vi "GlobalVariables.vi"() -> ()   [LabVIEW 2011]
uses:
  Controls/PC Cluster.ctl
  Controls/Device Cluster.ctl
  Controls/MFC Cluster.ctl
  Controls/RTPC Cluster.ctl
  Controls/GP275 Cluster.ctl
  Controls/BAR Cluster.ctl
  Controls/EZ-ZONE Input Cluster.ctl
  Controls/EZ-ZONE Output Cluster.ctl
  Controls/GP354 Cluster.ctl
  Controls/DNet StatusRegister Cluster.ctl
  Controls/DNet Status Cluster.ctl
  Controls/DNet CommandRegister Cluster.ctl
  Controls/TurboMotor Response Cluster.ctl
  Controls/TurboMotor Command Cluster.ctl
panel:
  out "Loop Started":bool
  out "Loop Running":bool
  in  "Write Enabled":bool
  in  "Reinitialize?":bool
  in  "Tab Control":T1(tab)
  in  "DNet CommandRegister Buffer":bool[](array[boolean])
  in  "DNet ScanCounter Strings":string[](array[string])
  out "DNet LCD Array":string[](array[string])
  in  "DNet CommandRegister Array":T2[](array[typedef])=[{"Run"=FALSE, "Fault"=FALSE, "DisableNetowrk"=FALSE, "HaltScanner"=FALSE, "Reset"=FALSE}, {"Run"=FALSE, "Fault"=FALSE, "DisableNetowrk"=FALSE, "HaltScanner"=FALSE, "Reset"=FALSE}, {"Run"=FALSE, "Fault"=FALSE, "DisableNetowrk"=FALSE, "HaltScanner"=FALSE, "Reset"=FALSE}, {"Run"=FALSE, "Fault"=FALSE, "DisableNetowrk"=FALSE, "HaltScanner"=FALSE, "Reset"=FALSE}]
  in  "DNet Status Array":T3[](array[typedef])
  out "DNet StatusRegister Array":T4[](array[typedef])
  in  "DNet StatusRegister Strings":string[](array[string])
  in  "DNet Status Strings":string[](array[string])
  in  "DNet CommandRegister Strings":string[](array[string])
  in  "Dnet Input Bytes":u8[](array[numeric])
  out "Dnet Output Bytes":u8[](array[numeric])
  out "Dnet Map Strings":string[][](array[string])=[["Dnet", "Node", "Type", "ID Number", "SCCM", "FullScale", "Input Bytes", "Output Bytes", "Input Start Location", "Output Start Location"], ["A", "1", "MFC", "1", "200", "24576", "8", "2", "0", "0"], ["A", "2", "MFC", "44", "2000", "24576", "8", "2", "8", "2"], ["A", "3", "MFC", "45", "200", "24576", "8", "2", "16", "4"], ["A", "4", "PC", "10", "2000", "0", "8", "2", "24", "6"], ["A", "5", "MFC", "2", "200", "24576", "8", "2", "32", "8"], ["A", "6", "MFC", "46", "2000", "24576", "8", "2", "40", "10"], ["A", "7", "MFC", "47", "200", "24576", "8", "2", "48", "12"], ["A", "8", "PC", "11", "2000", "0", "8", "2", "56", "14"], ["A", "9", "MFC", "3", "1000", "24576", "8", "2", "64", "16"], ["A", "10", "PC", "12", "1000", "0", "8", "2", "72", "18"], ["A", "11", "UNITMFC", "4", "500", "0", "8", "2", "80", "20"], ["A", "12", "PC", "13", "500", "0", "8", "2", "88", "22"], ["A", "13", "MFC", "5", "100", "24576", "8", "2", "96", "24"], ["A", "14", "MFC", "48", "1000", "24576", "8", "2", "104", "26"], ["A", "15", "MFC", "49", "100", "24576", "8", "2", "112", "28"], ["A", "16", "PC", "14", "1000", "0", "8", "2", "120", "30"], ["A", "17", "MFC", "6", "100", "24576", "8", "2", "128", "32"], ["A", "19", "MFC", "51", "100", "24576", "8", "2", "136", "34"], ["A", "20", "PC", "15", "1000", "0", "8", "2", "144", "36"], ["A", "21", "MFC", "7", "100", "24576", "8", "2", "152", "38"], ["A", "23", "MFC", "53", "100", "24576", "8", "2", "160", "40"], ["A", "24", "PC", "16", "1000", "0", "8", "2", "168", "42"], ["A", "25", "MFC", "8", "200", "24576", "8", "2", "176", "44"], ["A", "27", "MFC", "55", "200", "24576", "8", "2", "184", "46"], ["A", "28", "PC", "17", "1000", "0", "8", "2", "192", "48"], ["A", "31", "MFC", "37", "100", "24576", "8", "2", "200", "50"], ["A", "32", "MFC", "56", "500", "24576", "8", "2", "208", "52"], ["A", "37", "MFC", "52", "1000", "24576", "8", "2", "216", "54"], ["A", "42", "MFC", "42", "500", "24576", "8", "2", "224", "56"], ["A", "48", "BAR", "90", "0", "0", "3", "0", "232", "58"], ["A", "49", "RTPC", "29", "5000", "24576", "8", "3", "235", "58"], ["A", "50", "UNITMFC", "50", "1000", "24576", "8", "2", "243", "61"], ["A", "51", "UNITMFC", "54", "2000", "24576", "8", "2", "251", "63"], ["A", "53", "RTPC", "27", "5000", "24576", "8", "3", "259", "65"], ["A", "54", "RTPC", "28", "5000", "24576", "8", "3", "267", "68"], ["A", "55", "MFC", "57", "1000", "24576", "8", "2", "275", "71"], ["A", "56", "MFC", "41", "10", "24576", "8", "2", "283", "73"], ["A", "61", "BAR", "91", "0", "0", "3", "0", "291", "75"], ["B", "1", "MFC", "78", "2000", "24576", "8", "2", "294", "75"], ["B", "2", "MFC", "79", "2000", "24576", "8", "2", "302", "77"], ["B", "3", "MFC", "80", "2000", "24576", "8", "2", "310", "79"], ["B", "4", "MFC", "83", "20000", "24576", "8", "2", "318", "81"], ["B", "5", "MFC", "81", "20000", "24576", "8", "2", "326", "83"], ["B", "6", "MFC", "82", "20000", "24576", "8", "2", "334", "85"], ["B", "8", "MFC", "68", "2000", "24576", "8", "2", "342", "87"], ["B", "9", "MFC", "85", "1000", "24576", "8", "2", "350", "89"], ["B", "10", "MFC", "69", "2000", "24576", "8", "2", "358", "91"], ["B", "11", "MFC", "86", "2000", "24576", "8", "2", "366", "93"], ["B", "12", "MFC", "70", "500", "24576", "8", "2", "374", "95"], ["B", "13", "MFC", "73", "1000", "24576", "8", "2", "382", "97"], ["B", "14", "MFC", "74", "1000", "24576", "8", "2", "390", "99"], ["B", "15", "MFC", "75", "5000", "24576", "8", "2", "398", "101"], ["B", "16", "BAR", "92", "0", "0", "3", "0", "406", "103"], ["B", "21", "GP354", "0", "0", "0", "3", "1", "409", "103"], ["B", "22", "GP275", "0", "0", "0", "5", "0", "412", "104"], ["C", "1", "FESTO", "1", "0", "0", "2", "2", "417", "104"], ["C", "2", "FESTO", "2", "0", "0", "2", "2", "419", "106"], ["C", "3", "FESTO", "3", "0", "0", "2", "2", "421", "108"], ["C", "4", "FESTO", "4", "0", "0", "2", "2", "423", "110"], ["C", "5", "FESTO", "5", "0", "0", "2", "2", "425", "112"], ["C", "6", "FESTO", "6", "0", "0", "2", "2", "427", "114"], ["C", "7", "FESTO", "7", "0", "0", "2", "2", "429", "116"], ["C", "8", "FESTO", "8", "0", "0", "2", "2", "431", "118"]]
  in  "Dnet Input Strings":string[](array[string])=["Dnet_A_N01_POL_I.Data", "Dnet_A_N01_POL_I.Data1", "Dnet_A_N01_POL_I.Data2", "Dnet_A_N01_POL_I.ExtendedData", "Dnet_A_N01_POL_I.ExtendedData1", "Dnet_A_N01_POL_I.ExtendedData2", "Dnet_A_N01_POL_I.ExtendedData3", "Dnet_A_N01_POL_I.ExtendedData4", "Dnet_A_N02_POL_I.Data", "Dnet_A_N02_POL_I.Data1", "Dnet_A_N02_POL_I.Data2", "Dnet_A_N02_POL_I.ExtendedData", "Dnet_A_N02_POL_I.ExtendedData1", "Dnet_A_N02_POL_I.ExtendedData2", "Dnet_A_N02_POL_I.ExtendedData3", "Dnet_A_N02_POL_I.ExtendedData4", "Dnet_A_N03_POL_I.Data", "Dnet_A_N03_POL_I.Data1", "Dnet_A_N03_POL_I.Data2", "Dnet_A_N03_POL_I.ExtendedData", "Dnet_A_N03_POL_I.ExtendedData1", "Dnet_A_N03_POL_I.ExtendedData2", "Dnet_A_N03_POL_I.ExtendedData3", "Dnet_A_N03_POL_I.ExtendedData4", "Dnet_A_N04_POL_I.Data", "Dnet_A_N04_POL_I.Data1", "Dnet_A_N04_POL_I.Data2", "Dnet_A_N04_POL_I.ExtendedData", "Dnet_A_N04_POL_I.ExtendedData1", "Dnet_A_N04_POL_I.ExtendedData2", "Dnet_A_N04_POL_I.ExtendedData3", "Dnet_A_N04_POL_I.ExtendedData4", "Dnet_A_N05_POL_I.Data", "Dnet_A_N05_POL_I.Data1", "Dnet_A_N05_POL_I.Data2", "Dnet_A_N05_POL_I.ExtendedData", "Dnet_A_N05_POL_I.ExtendedData1", "Dnet_A_N05_POL_I.ExtendedData2", "Dnet_A_N05_POL_I.ExtendedData3", "Dnet_A_N05_POL_I.ExtendedData4", "Dnet_A_N06_POL_I.Data", "Dnet_A_N06_POL_I.Data1", "Dnet_A_N06_POL_I.Data2", "Dnet_A_N06_POL_I.ExtendedData", "Dnet_A_N06_POL_I.ExtendedData1", "Dnet_A_N06_POL_I.ExtendedData2", "Dnet_A_N06_POL_I.ExtendedData3", "Dnet_A_N06_POL_I.ExtendedData4", "Dnet_A_N07_POL_I.Data", "Dnet_A_N07_POL_I.Data1", "Dnet_A_N07_POL_I.Data2", "Dnet_A_N07_POL_I.ExtendedData", "Dnet_A_N07_POL_I.ExtendedData1", "Dnet_A_N07_POL_I.ExtendedData2", "Dnet_A_N07_POL_I.ExtendedData3", "Dnet_A_N07_POL_I.ExtendedData4", "Dnet_A_N08_POL_I.Data", "Dnet_A_N08_POL_I.Data1", "Dnet_A_N08_POL_I.Data2", "Dnet_A_N08_POL_I.ExtendedData", "Dnet_A_N08_POL_I.ExtendedData1", "Dnet_A_N08_POL_I.ExtendedData2", "Dnet_A_N08_POL_I.ExtendedData3", "Dnet_A_N08_POL_I.ExtendedData4", "Dnet_A_N09_POL_I.Data", "Dnet_A_N09_POL_I.Data1", "Dnet_A_N09_POL_I.Data2", "Dnet_A_N09_POL_I.ExtendedData", "Dnet_A_N09_POL_I.ExtendedData1", "Dnet_A_N09_POL_I.ExtendedData2", "Dnet_A_N09_POL_I.ExtendedData3", "Dnet_A_N09_POL_I.ExtendedData4", "Dnet_A_N10_POL_I.Data", "Dnet_A_N10_POL_I.Data1", "Dnet_A_N10_POL_I.Data2", "Dnet_A_N10_POL_I.ExtendedData", "Dnet_A_N10_POL_I.ExtendedData1", "Dnet_A_N10_POL_I.ExtendedData2", "Dnet_A_N10_POL_I.ExtendedData3", "Dnet_A_N10_POL_I.ExtendedData4", "Dnet_A_N11_POL_I.Data_x.Data_0", "Dnet_A_N11_POL_I.Data_x.Data_1", "Dnet_A_N11_POL_I.Data_x.Data_2", "Dnet_A_N11_POL_I.Data_x.Data_3", "Dnet_A_N11_POL_I.Data_x.Data_4", "Dnet_A_N11_POL_I.Data_x.Data_5", "Dnet_A_N11_POL_I.Data_x.Data_6", "Dnet_A_N11_POL_I.Data_x.Data_7", "Dnet_A_N12_POL_I.Data", "Dnet_A_N12_POL_I.Data1", "Dnet_A_N12_POL_I.Data2", "Dnet_A_N12_POL_I.ExtendedData", "Dnet_A_N12_POL_I.ExtendedData1", "Dnet_A_N12_POL_I.ExtendedData2", "Dnet_A_N12_POL_I.ExtendedData3", "Dnet_A_N12_POL_I.ExtendedData4", "Dnet_A_N13_POL_I.Data", "Dnet_A_N13_POL_I.Data1", "Dnet_A_N13_POL_I.Data2", "Dnet_A_N13_POL_I.ExtendedData", "Dnet_A_N13_POL_I.ExtendedData1", "Dnet_A_N13_POL_I.ExtendedData2", "Dnet_A_N13_POL_I.ExtendedData3", "Dnet_A_N13_POL_I.ExtendedData4", "Dnet_A_N14_POL_I.Data", "Dnet_A_N14_POL_I.Data1", "Dnet_A_N14_POL_I.Data2", "Dnet_A_N14_POL_I.ExtendedData", "Dnet_A_N14_POL_I.ExtendedData1", "Dnet_A_N14_POL_I.ExtendedData2", "Dnet_A_N14_POL_I.ExtendedData3", "Dnet_A_N14_POL_I.ExtendedData4", "Dnet_A_N15_POL_I.Data", "Dnet_A_N15_POL_I.Data1", "Dnet_A_N15_POL_I.Data2", "Dnet_A_N15_POL_I.ExtendedData", "Dnet_A_N15_POL_I.ExtendedData1", "Dnet_A_N15_POL_I.ExtendedData2", "Dnet_A_N15_POL_I.ExtendedData3", "Dnet_A_N15_POL_I.ExtendedData4", "Dnet_A_N16_POL_I.Data", "Dnet_A_N16_POL_I.Data1", "Dnet_A_N16_POL_I.Data2", "Dnet_A_N16_POL_I.ExtendedData", "Dnet_A_N16_POL_I.ExtendedData1", "Dnet_A_N16_POL_I.ExtendedData2", "Dnet_A_N16_POL_I.ExtendedData3", "Dnet_A_N16_POL_I.ExtendedData4", "Dnet_A_N17_POL_I.Data", "Dnet_A_N17_POL_I.Data1", "Dnet_A_N17_POL_I.Data2", "Dnet_A_N17_POL_I.ExtendedData", "Dnet_A_N17_POL_I.ExtendedData1", "Dnet_A_N17_POL_I.ExtendedData2", "Dnet_A_N17_POL_I.ExtendedData3", "Dnet_A_N17_POL_I.ExtendedData4", "Dnet_A_N19_POL_I.Data", "Dnet_A_N19_POL_I.Data1", "Dnet_A_N19_POL_I.Data2", "Dnet_A_N19_POL_I.ExtendedData", "Dnet_A_N19_POL_I.ExtendedData1", "Dnet_A_N19_POL_I.ExtendedData2", "Dnet_A_N19_POL_I.ExtendedData3", "Dnet_A_N19_POL_I.ExtendedData4", "Dnet_A_N20_POL_I.Data", "Dnet_A_N20_POL_I.Data1", "Dnet_A_N20_POL_I.Data2", "Dnet_A_N20_POL_I.ExtendedData", "Dnet_A_N20_POL_I.ExtendedData1", "Dnet_A_N20_POL_I.ExtendedData2", "Dnet_A_N20_POL_I.ExtendedData3", "Dnet_A_N20_POL_I.ExtendedData4", "Dnet_A_N21_POL_I.Data", "Dnet_A_N21_POL_I.Data1", "Dnet_A_N21_POL_I.Data2", "Dnet_A_N21_POL_I.ExtendedData", "Dnet_A_N21_POL_I.ExtendedData1", "Dnet_A_N21_POL_I.ExtendedData2", "Dnet_A_N21_POL_I.ExtendedData3", "Dnet_A_N21_POL_I.ExtendedData4", "Dnet_A_N23_POL_I.Data", "Dnet_A_N23_POL_I.Data1", "Dnet_A_N23_POL_I.Data2", "Dnet_A_N23_POL_I.ExtendedData", "Dnet_A_N23_POL_I.ExtendedData1", "Dnet_A_N23_POL_I.ExtendedData2", "Dnet_A_N23_POL_I.ExtendedData3", "Dnet_A_N23_POL_I.ExtendedData4", "Dnet_A_N24_POL_I.Data", "Dnet_A_N24_POL_I.Data1", "Dnet_A_N24_POL_I.Data2", "Dnet_A_N24_POL_I.ExtendedData", "Dnet_A_N24_POL_I.ExtendedData1", "Dnet_A_N24_POL_I.ExtendedData2", "Dnet_A_N24_POL_I.ExtendedData3", "Dnet_A_N24_POL_I.ExtendedData4", "Dnet_A_N25_POL_I.Data", "Dnet_A_N25_POL_I.Data1", "Dnet_A_N25_POL_I.Data2", "Dnet_A_N25_POL_I.ExtendedData", "Dnet_A_N25_POL_I.ExtendedData1", "Dnet_A_N25_POL_I.ExtendedData2", "Dnet_A_N25_POL_I.ExtendedData3", "Dnet_A_N25_POL_I.ExtendedData4", "Dnet_A_N27_POL_I.Data", "Dnet_A_N27_POL_I.Data1", "Dnet_A_N27_POL_I.Data2", "Dnet_A_N27_POL_I.ExtendedData", "Dnet_A_N27_POL_I.ExtendedData1", "Dnet_A_N27_POL_I.ExtendedData2", "Dnet_A_N27_POL_I.ExtendedData3", "Dnet_A_N27_POL_I.ExtendedData4", "Dnet_A_N28_POL_I.Data", "Dnet_A_N28_POL_I.Data1", "Dnet_A_N28_POL_I.Data2", "Dnet_A_N28_POL_I.ExtendedData", "Dnet_A_N28_POL_I.ExtendedData1", "Dnet_A_N28_POL_I.ExtendedData2", "Dnet_A_N28_POL_I.ExtendedData3", "Dnet_A_N28_POL_I.ExtendedData4", "Dnet_A_N31_POL_I.Data", "Dnet_A_N31_POL_I.Data1", "Dnet_A_N31_POL_I.Data2", "Dnet_A_N31_POL_I.ExtendedData", "Dnet_A_N31_POL_I.ExtendedData1", "Dnet_A_N31_POL_I.ExtendedData2", "Dnet_A_N31_POL_I.ExtendedData3", "Dnet_A_N31_POL_I.ExtendedData4", "Dnet_A_N32_POL_I.Data", "Dnet_A_N32_POL_I.Data1", "Dnet_A_N32_POL_I.Data2", "Dnet_A_N32_POL_I.ExtendedData", "Dnet_A_N32_POL_I.ExtendedData1", "Dnet_A_N32_POL_I.ExtendedData2", "Dnet_A_N32_POL_I.ExtendedData3", "Dnet_A_N32_POL_I.ExtendedData4", "Dnet_A_N37_POL_I.Data_x.Data_0", "Dnet_A_N37_POL_I.Data_x.Data_1", "Dnet_A_N37_POL_I.Data_x.Data_2", "Dnet_A_N37_POL_I.Data_x.Data_3", "Dnet_A_N37_POL_I.Data_x.Data_4", "Dnet_A_N37_POL_I.Data_x.Data_5", "Dnet_A_N37_POL_I.Data_x.Data_6", "Dnet_A_N37_POL_I.Data_x.Data_7", "Dnet_A_N42_POL_I.Data", "Dnet_A_N42_POL_I.Data1", "Dnet_A_N42_POL_I.Data2", "Dnet_A_N42_POL_I.ExtendedData", "Dnet_A_N42_POL_I.ExtendedData1", "Dnet_A_N42_POL_I.ExtendedData2", "Dnet_A_N42_POL_I.ExtendedData3", "Dnet_A_N42_POL_I.ExtendedData4", "Dnet_A_N48_POL_I.Data_x.Data_0", "Dnet_A_N48_POL_I.Data_x.Data_1", "Dnet_A_N48_POL_I.Data_x.Data_2", "Dnet_A_N49_POL_I.Data", "Dnet_A_N49_POL_I.Data1", "Dnet_A_N49_POL_I.Data2", "Dnet_A_N49_POL_I.ExtendedData", "Dnet_A_N49_POL_I.ExtendedData1", "Dnet_A_N49_POL_I.ExtendedData2", "Dnet_A_N49_POL_I.ExtendedData3", "Dnet_A_N49_POL_I.ExtendedData4", "Dnet_A_N50_POL_I.Data_x.Data_0", "Dnet_A_N50_POL_I.Data_x.Data_1", "Dnet_A_N50_POL_I.Data_x.Data_2", "Dnet_A_N50_POL_I.Data_x.Data_3", "Dnet_A_N50_POL_I.Data_x.Data_4", "Dnet_A_N50_POL_I.Data_x.Data_5", "Dnet_A_N50_POL_I.Data_x.Data_6", "Dnet_A_N50_POL_I.Data_x.Data_7", "Dnet_A_N51_POL_I.Data_x.Data_0", "Dnet_A_N51_POL_I.Data_x.Data_1", "Dnet_A_N51_POL_I.Data_x.Data_2", "Dnet_A_N51_POL_I.Data_x.Data_3", "Dnet_A_N51_POL_I.Data_x.Data_4", "Dnet_A_N51_POL_I.Data_x.Data_5", "Dnet_A_N51_POL_I.Data_x.Data_6", "Dnet_A_N51_POL_I.Data_x.Data_7", "Dnet_A_N53_POL_I.Data", "Dnet_A_N53_POL_I.Data1", "Dnet_A_N53_POL_I.Data2", "Dnet_A_N53_POL_I.ExtendedData", "Dnet_A_N53_POL_I.ExtendedData1", "Dnet_A_N53_POL_I.ExtendedData2", "Dnet_A_N53_POL_I.ExtendedData3", "Dnet_A_N53_POL_I.ExtendedData4", "Dnet_A_N54_POL_I.Data", "Dnet_A_N54_POL_I.Data1", "Dnet_A_N54_POL_I.Data2", "Dnet_A_N54_POL_I.ExtendedData", "Dnet_A_N54_POL_I.ExtendedData1", "Dnet_A_N54_POL_I.ExtendedData2", "Dnet_A_N54_POL_I.ExtendedData3", "Dnet_A_N54_POL_I.ExtendedData4", "Dnet_A_N55_POL_I.Data", "Dnet_A_N55_POL_I.Data1", "Dnet_A_N55_POL_I.Data2", "Dnet_A_N55_POL_I.ExtendedData", "Dnet_A_N55_POL_I.ExtendedData1", "Dnet_A_N55_POL_I.ExtendedData2", "Dnet_A_N55_POL_I.ExtendedData3", "Dnet_A_N55_POL_I.ExtendedData4", "Dnet_A_N56_POL_I.Data", "Dnet_A_N56_POL_I.Data1", "Dnet_A_N56_POL_I.Data2", "Dnet_A_N56_POL_I.ExtendedData", "Dnet_A_N56_POL_I.ExtendedData1", "Dnet_A_N56_POL_I.ExtendedData2", "Dnet_A_N56_POL_I.ExtendedData3", "Dnet_A_N56_POL_I.ExtendedData4", "Dnet_A_N61_POL_I.Data_x.Data_0", "Dnet_A_N61_POL_I.Data_x.Data_1", "Dnet_A_N61_POL_I.Data_x.Data_2", "Dnet_B_N01_POL_I.Data", "Dnet_B_N01_POL_I.Data1", "Dnet_B_N01_POL_I.Data2", "Dnet_B_N01_POL_I.ExtendedData", "Dnet_B_N01_POL_I.ExtendedData1", "Dnet_B_N01_POL_I.ExtendedData2", "Dnet_B_N01_POL_I.ExtendedData3", "Dnet_B_N01_POL_I.ExtendedData4", "Dnet_B_N02_POL_I.Data", "Dnet_B_N02_POL_I.Data1", "Dnet_B_N02_POL_I.Data2", "Dnet_B_N02_POL_I.ExtendedData", "Dnet_B_N02_POL_I.ExtendedData1", "Dnet_B_N02_POL_I.ExtendedData2", "Dnet_B_N02_POL_I.ExtendedData3", "Dnet_B_N02_POL_I.ExtendedData4", "Dnet_B_N03_POL_I.Data", "Dnet_B_N03_POL_I.Data1", "Dnet_B_N03_POL_I.Data2", "Dnet_B_N03_POL_I.ExtendedData", "Dnet_B_N03_POL_I.ExtendedData1", "Dnet_B_N03_POL_I.ExtendedData2", "Dnet_B_N03_POL_I.ExtendedData3", "Dnet_B_N03_POL_I.ExtendedData4", "Dnet_B_N04_POL_I.Data", "Dnet_B_N04_POL_I.Data1", "Dnet_B_N04_POL_I.Data2", "Dnet_B_N04_POL_I.ExtendedData", "Dnet_B_N04_POL_I.ExtendedData1", "Dnet_B_N04_POL_I.ExtendedData2", "Dnet_B_N04_POL_I.ExtendedData3", "Dnet_B_N04_POL_I.ExtendedData4", "Dnet_B_N05_POL_I.Data", "Dnet_B_N05_POL_I.Data1", "Dnet_B_N05_POL_I.Data2", "Dnet_B_N05_POL_I.ExtendedData", "Dnet_B_N05_POL_I.ExtendedData1", "Dnet_B_N05_POL_I.ExtendedData2", "Dnet_B_N05_POL_I.ExtendedData3", "Dnet_B_N05_POL_I.ExtendedData4", "Dnet_B_N06_POL_I.Data", "Dnet_B_N06_POL_I.Data1", "Dnet_B_N06_POL_I.Data2", "Dnet_B_N06_POL_I.ExtendedData", "Dnet_B_N06_POL_I.ExtendedData1", "Dnet_B_N06_POL_I.ExtendedData2", "Dnet_B_N06_POL_I.ExtendedData3", "Dnet_B_N06_POL_I.ExtendedData4", "Dnet_B_N08_POL_I.Data", "Dnet_B_N08_POL_I.Data1", "Dnet_B_N08_POL_I.Data2", "Dnet_B_N08_POL_I.ExtendedData", "Dnet_B_N08_POL_I.ExtendedData1", "Dnet_B_N08_POL_I.ExtendedData2", "Dnet_B_N08_POL_I.ExtendedData3", "Dnet_B_N08_POL_I.ExtendedData4", "Dnet_B_N09_POL_I.Data", "Dnet_B_N09_POL_I.Data1", "Dnet_B_N09_POL_I.Data2", "Dnet_B_N09_POL_I.ExtendedData", "Dnet_B_N09_POL_I.ExtendedData1", "Dnet_B_N09_POL_I.ExtendedData2", "Dnet_B_N09_POL_I.ExtendedData3", "Dnet_B_N09_POL_I.ExtendedData4", "Dnet_B_N10_POL_I.Data", "Dnet_B_N10_POL_I.Data1", "Dnet_B_N10_POL_I.Data2", "Dnet_B_N10_POL_I.ExtendedData", "Dnet_B_N10_POL_I.ExtendedData1", "Dnet_B_N10_POL_I.ExtendedData2", "Dnet_B_N10_POL_I.ExtendedData3", "Dnet_B_N10_POL_I.ExtendedData4", "Dnet_B_N11_POL_I.Data", "Dnet_B_N11_POL_I.Data1", "Dnet_B_N11_POL_I.Data2", "Dnet_B_N11_POL_I.ExtendedData", "Dnet_B_N11_POL_I.ExtendedData1", "Dnet_B_N11_POL_I.ExtendedData2", "Dnet_B_N11_POL_I.ExtendedData3", "Dnet_B_N11_POL_I.ExtendedData4", "Dnet_B_N12_POL_I.Data", "Dnet_B_N12_POL_I.Data1", "Dnet_B_N12_POL_I.Data2", "Dnet_B_N12_POL_I.ExtendedData", "Dnet_B_N12_POL_I.ExtendedData1", "Dnet_B_N12_POL_I.ExtendedData2", "Dnet_B_N12_POL_I.ExtendedData3", "Dnet_B_N12_POL_I.ExtendedData4", "Dnet_B_N13_POL_I.Data", "Dnet_B_N13_POL_I.Data1", "Dnet_B_N13_POL_I.Data2", "Dnet_B_N13_POL_I.ExtendedData", "Dnet_B_N13_POL_I.ExtendedData1", "Dnet_B_N13_POL_I.ExtendedData2", "Dnet_B_N13_POL_I.ExtendedData3", "Dnet_B_N13_POL_I.ExtendedData4", "Dnet_B_N14_POL_I.Data", "Dnet_B_N14_POL_I.Data1", "Dnet_B_N14_POL_I.Data2", "Dnet_B_N14_POL_I.ExtendedData", "Dnet_B_N14_POL_I.ExtendedData1", "Dnet_B_N14_POL_I.ExtendedData2", "Dnet_B_N14_POL_I.ExtendedData3", "Dnet_B_N14_POL_I.ExtendedData4", "Dnet_B_N15_POL_I.Data", "Dnet_B_N15_POL_I.Data1", "Dnet_B_N15_POL_I.Data2", "Dnet_B_N15_POL_I.ExtendedData", "Dnet_B_N15_POL_I.ExtendedData1", "Dnet_B_N15_POL_I.ExtendedData2", "Dnet_B_N15_POL_I.ExtendedData3", "Dnet_B_N15_POL_I.ExtendedData4", "Dnet_B_N16_POL_I.Data_x.Data_0", "Dnet_B_N16_POL_I.Data_x.Data_1", "Dnet_B_N16_POL_I.Data_x.Data_2", "Dnet_B_N21_POL_I.Data_x.Data_0", "Dnet_B_N21_POL_I.Data_x.Data_1", "Dnet_B_N21_POL_I.Data_x.Data_2", "Dnet_B_N22_POL_I.Data_x.Data_0", "Dnet_B_N22_POL_I.Data_x.Data_1", "Dnet_B_N22_POL_I.Data_x.Data_2", "Dnet_B_N22_POL_I.Data_x.Data_3", "Dnet_B_N22_POL_I.Data_x.Data_4", "Dnet_C_N01_POL_I.Data", "Dnet_C_N01_STB_I.Data", "Dnet_C_N02_POL_I.Data_x.Data_0", "Dnet_C_N02_POL_I.Data_x.Data_1", "Dnet_C_N03_POL_I.Data_x.Data_0", "Dnet_C_N03_POL_I.Data_x.Data_1", "Dnet_C_N04_POL_I.Data_x.Data_0", "Dnet_C_N04_POL_I.Data_x.Data_1", "Dnet_C_N05_POL_I.Data_x.Data_0", "Dnet_C_N05_POL_I.Data_x.Data_1", "Dnet_C_N06_POL_I.Data_x.Data_0", "Dnet_C_N06_POL_I.Data_x.Data_1", "Dnet_C_N07_POL_I.Data_x.Data_0", "Dnet_C_N07_POL_I.Data_x.Data_1", "Dnet_C_N08_POL_I.Data_x.Data_0", "Dnet_C_N08_POL_I.Data_x.Data_1"]
  in  "Dnet Output Strings":string[](array[string])=["Dnet_A_N01_POL_O.Data_x.Data_0", "Dnet_A_N01_POL_O.Data_x.Data_1", "Dnet_A_N02_POL_O.Data_x.Data_0", "Dnet_A_N02_POL_O.Data_x.Data_1", "Dnet_A_N03_POL_O.Data_x.Data_0", "Dnet_A_N03_POL_O.Data_x.Data_1", "Dnet_A_N04_POL_O.Data_x.Data_0", "Dnet_A_N04_POL_O.Data_x.Data_1", "Dnet_A_N05_POL_O.Data_x.Data_0", "Dnet_A_N05_POL_O.Data_x.Data_1", "Dnet_A_N06_POL_O.Data_x.Data_0", "Dnet_A_N06_POL_O.Data_x.Data_1", "Dnet_A_N07_POL_O.Data_x.Data_0", "Dnet_A_N07_POL_O.Data_x.Data_1", "Dnet_A_N08_POL_O.Data_x.Data_0", "Dnet_A_N08_POL_O.Data_x.Data_1", "Dnet_A_N09_POL_O.Data_x.Data_0", "Dnet_A_N09_POL_O.Data_x.Data_1", "Dnet_A_N10_POL_O.Data_x.Data_0", "Dnet_A_N10_POL_O.Data_x.Data_1", "Dnet_A_N11_POL_O.Data_x.Data_0", "Dnet_A_N11_POL_O.Data_x.Data_1", "Dnet_A_N12_POL_O.Data_x.Data_0", "Dnet_A_N12_POL_O.Data_x.Data_1", "Dnet_A_N13_POL_O.Data_x.Data_0", "Dnet_A_N13_POL_O.Data_x.Data_1", "Dnet_A_N14_POL_O.Data_x.Data_0", "Dnet_A_N14_POL_O.Data_x.Data_1", "Dnet_A_N15_POL_O.Data_x.Data_0", "Dnet_A_N15_POL_O.Data_x.Data_1", "Dnet_A_N16_POL_O.Data_x.Data_0", "Dnet_A_N16_POL_O.Data_x.Data_1", "Dnet_A_N17_POL_O.Data_x.Data_0", "Dnet_A_N17_POL_O.Data_x.Data_1", "Dnet_A_N19_POL_O.Data_x.Data_0", "Dnet_A_N19_POL_O.Data_x.Data_1", "Dnet_A_N20_POL_O.Data_x.Data_0", "Dnet_A_N20_POL_O.Data_x.Data_1", "Dnet_A_N21_POL_O.Data_x.Data_0", "Dnet_A_N21_POL_O.Data_x.Data_1", "Dnet_A_N23_POL_O.Data_x.Data_0", "Dnet_A_N23_POL_O.Data_x.Data_1", "Dnet_A_N24_POL_O.Data_x.Data_0", "Dnet_A_N24_POL_O.Data_x.Data_1", "Dnet_A_N25_POL_O.Data_x.Data_0", "Dnet_A_N25_POL_O.Data_x.Data_1", "Dnet_A_N27_POL_O.Data_x.Data_0", "Dnet_A_N27_POL_O.Data_x.Data_1", "Dnet_A_N28_POL_O.Data_x.Data_0", "Dnet_A_N28_POL_O.Data_x.Data_1", "Dnet_A_N31_POL_O.Data_x.Data_0", "Dnet_A_N31_POL_O.Data_x.Data_1", "Dnet_A_N32_POL_O.Data_x.Data_0", "Dnet_A_N32_POL_O.Data_x.Data_1", "Dnet_A_N37_POL_O.Data_x.Data_0", "Dnet_A_N37_POL_O.Data_x.Data_1", "Dnet_A_N42_POL_O.Data_x.Data_0", "Dnet_A_N42_POL_O.Data_x.Data_1", "Dnet_A_N49_POL_O.Data", "Dnet_A_N49_POL_O.Data1", "Dnet_A_N49_POL_O.ExtendedData", "Dnet_A_N50_POL_O.Data_x.Data_0", "Dnet_A_N50_POL_O.Data_x.Data_1", "Dnet_A_N51_POL_O.Data_x.Data_0", "Dnet_A_N51_POL_O.Data_x.Data_1", "Dnet_A_N53_POL_O.Data", "Dnet_A_N53_POL_O.Data1", "Dnet_A_N53_POL_O.ExtendedData", "Dnet_A_N54_POL_O.Data", "Dnet_A_N54_POL_O.Data1", "Dnet_A_N54_POL_O.ExtendedData", "Dnet_A_N55_POL_O.Data_x.Data_0", "Dnet_A_N55_POL_O.Data_x.Data_1", "Dnet_A_N56_POL_O.Data_x.Data_0", "Dnet_A_N56_POL_O.Data_x.Data_1", "Dnet_B_N01_POL_O.Data_x.Data_0", "Dnet_B_N01_POL_O.Data_x.Data_1", "Dnet_B_N02_POL_O.Data_x.Data_0", "Dnet_B_N02_POL_O.Data_x.Data_1", "Dnet_B_N03_POL_O.Data_x.Data_0", "Dnet_B_N03_POL_O.Data_x.Data_1", "Dnet_B_N04_POL_O.Data_x.Data_0", "Dnet_B_N04_POL_O.Data_x.Data_1", "Dnet_B_N05_POL_O.Data_x.Data_0", "Dnet_B_N05_POL_O.Data_x.Data_1", "Dnet_B_N06_POL_O.Data_x.Data_0", "Dnet_B_N06_POL_O.Data_x.Data_1", "Dnet_B_N08_POL_O.Data_x.Data_0", "Dnet_B_N08_POL_O.Data_x.Data_1", "Dnet_B_N09_POL_O.Data_x.Data_0", "Dnet_B_N09_POL_O.Data_x.Data_1", "Dnet_B_N10_POL_O.Data_x.Data_0", "Dnet_B_N10_POL_O.Data_x.Data_1", "Dnet_B_N11_POL_O.Data_x.Data_0", "Dnet_B_N11_POL_O.Data_x.Data_1", "Dnet_B_N12_POL_O.Data_x.Data_0", "Dnet_B_N12_POL_O.Data_x.Data_1", "Dnet_B_N13_POL_O.Data_x.Data_0", "Dnet_B_N13_POL_O.Data_x.Data_1", "Dnet_B_N14_POL_O.Data_x.Data_0", "Dnet_B_N14_POL_O.Data_x.Data_1", "Dnet_B_N15_POL_O.Data_x.Data_0", "Dnet_B_N15_POL_O.Data_x.Data_1", "Dnet_B_N21_POL_O.Data", "Dnet_C_N01_POL_O.Data_x.Data_0", "Dnet_C_N01_POL_O.Data_x.Data_1", "Dnet_C_N02_POL_O.Data_x.Data_0", "Dnet_C_N02_POL_O.Data_x.Data_1", "Dnet_C_N03_POL_O.Data_x.Data_0", "Dnet_C_N03_POL_O.Data_x.Data_1", "Dnet_C_N04_POL_O.Data_x.Data_0", "Dnet_C_N04_POL_O.Data_x.Data_1", "Dnet_C_N05_POL_O.Data_x.Data_0", "Dnet_C_N05_POL_O.Data_x.Data_1", "Dnet_C_N06_POL_O.Data_x.Data_0", "Dnet_C_N06_POL_O.Data_x.Data_1", "Dnet_C_N07_POL_O.Data_x.Data_0", "Dnet_C_N07_POL_O.Data_x.Data_1", "Dnet_C_N08_POL_O.Data_x.Data_0", "Dnet_C_N08_POL_O.Data_x.Data_1"]
  in  "Ain":dbl[](array[numeric])
  in  "Aout":i16[](array[numeric])
  in  "Ain1 Strings":string[](array[string])=["Local_5_I.Ch0Data", "Local_5_I.Ch1Data", "Local_5_I.Ch2Data", "Local_5_I.Ch3Data", "Local_5_I.Ch4Data", "Local_5_I.Ch5Data", "Local_5_I.Ch6Data", "Local_5_I.Ch7Data", "Local_5_I.Ch8Data", "Local_5_I.Ch9Data", "Local_5_I.Ch10Data", "Local_5_I.Ch11Data", "Local_5_I.Ch12Data", "Local_5_I.Ch13Data", "Local_5_I.Ch14Data", "Local_5_I.Ch15Data"]
  in  "Ain2 Strings":string[](array[string])=["Local_6_I.Ch0Data", "Local_6_I.Ch1Data", "Local_6_I.Ch2Data", "Local_6_I.Ch3Data", "Local_6_I.Ch4Data", "Local_6_I.Ch5Data", "Local_6_I.Ch6Data", "Local_6_I.Ch7Data", "Local_6_I.Ch8Data", "Local_6_I.Ch9Data", "Local_6_I.Ch10Data", "Local_6_I.Ch11Data", "Local_6_I.Ch12Data", "Local_6_I.Ch13Data", "Local_6_I.Ch14Data", "Local_6_I.Ch15Data"]
  in  "Dout Strings":string[](array[string])=["Local_10_O.Data"]
  in  "Din Strings":string[](array[string])=["Local_8_I.Data", "Local_9_I.Data", "Local_10_I.Data"]
  in  "Din1":bool[](array[boolean])=[FALSE, FALSE, FALSE, FALSE, FALSE, FALSE, FALSE, FALSE, FALSE, FALSE, FALSE, FALSE, FALSE, FALSE, FALSE, FALSE, FALSE, FALSE, FALSE, FALSE, FALSE, FALSE, FALSE, FALSE, FALSE, FALSE, FALSE, FALSE, FALSE, FALSE, FALSE, FALSE]
  in  "Dout":bool[](array[boolean])=[FALSE, FALSE, FALSE, FALSE, FALSE, FALSE, FALSE, FALSE, FALSE, FALSE, FALSE, FALSE, FALSE, FALSE, FALSE, FALSE, FALSE, FALSE, FALSE, FALSE, FALSE, FALSE, FALSE, FALSE, FALSE, FALSE, FALSE, FALSE, FALSE, FALSE, FALSE, FALSE]
  in  "Din2":bool[](array[boolean])=[FALSE, FALSE, FALSE, FALSE, FALSE, FALSE, FALSE, FALSE, FALSE, FALSE, FALSE, FALSE, FALSE, FALSE, FALSE, FALSE, FALSE, FALSE, FALSE, FALSE, FALSE, FALSE, FALSE, FALSE, FALSE, FALSE, FALSE, FALSE, FALSE, FALSE, FALSE, FALSE]
  in  "Valve Strings 2":string[](array[string])=["Valve_x.Valve_000", "Valve_x.Valve_001", "Valve_x.Valve_002", "Valve_x.Valve_003", "Valve_x.Valve_004", "Valve_x.Valve_005", "Valve_x.Valve_006", "Valve_x.Valve_007", "Valve_x.Valve_008", "Valve_x.Valve_009", "Valve_x.Valve_010", "Valve_x.Valve_011", "Valve_x.Valve_012", "Valve_x.Valve_013", "Valve_x.Valve_014", "Valve_x.Valve_015", "Valve_x.Valve_016", "Valve_x.Valve_017", "Valve_x.Valve_018", "Valve_x.Valve_019", "Valve_x.Valve_020", "Valve_x.Valve_021", "Valve_x.Valve_022", "Valve_x.Valve_023", "Valve_x.Valve_024", "Valve_x.Valve_025", "Valve_x.Valve_026", "Valve_x.Valve_027", "Valve_x.Valve_028", "Valve_x.Valve_029", "Valve_x.Valve_030", "Valve_x.Valve_031", "Valve_x.Valve_032", "Valve_x.Valve_033", "Valve_x.Valve_034", "Valve_x.Valve_035", "Valve_x.Valve_036", "Valve_x.Valve_037", "Valve_x.Valve_038", "Valve_x.Valve_039", "Valve_x.Valve_040", "Valve_x.Valve_041", "Valve_x.Valve_042", "Valve_x.Valve_043", "Valve_x.Valve_044", "Valve_x.Valve_045", "Valve_x.Valve_046", "Valve_x.Valve_047", "Valve_x.Valve_048", "Valve_x.Valve_049", "Valve_x.Valve_050", "Valve_x.Valve_051", "Valve_x.Valve_052", "Valve_x.Valve_053", "Valve_x.Valve_054", "Valve_x.Valve_055", "Valve_x.Valve_056", "Valve_x.Valve_057", "Valve_x.Valve_058", "Valve_x.Valve_059", "Valve_x.Valve_060", "Valve_x.Valve_061", "Valve_x.Valve_062", "Valve_x.Valve_063", "Valve_x.Valve_064", "Valve_x.Valve_065", "Valve_x.Valve_066", "Valve_x.Valve_067", "Valve_x.Valve_068", "Valve_x.Valve_069", "Valve_x.Valve_070", "Valve_x.Valve_071", "Valve_x.Valve_072", "Valve_x.Valve_073", "Valve_x.Valve_074", "Valve_x.Valve_075", "Valve_x.Valve_076", "Valve_x.Valve_077", "Valve_x.Valve_078", "Valve_x.Valve_079", "Valve_x.Valve_080", "Valve_x.Valve_081", "Valve_x.Valve_082", "Valve_x.Valve_083", "Valve_x.Valve_084", "Valve_x.Valve_085", "Valve_x.Valve_086", "Valve_x.Valve_087", "Valve_x.Valve_088", "Valve_x.Valve_089", "Valve_x.Valve_090", "Valve_x.Valve_091", "Valve_x.Valve_092", "Valve_x.Valve_093", "Valve_x.Valve_094", "Valve_x.Valve_095", "Valve_x.Valve_096", "Valve_x.Valve_097", "Valve_x.Valve_098", "Valve_x.Valve_099", "Valve_x.Valve_100", "Valve_x.Valve_101", "Valve_x.Valve_102", "Valve_x.Valve_103", "Valve_x.Valve_104", "Valve_x.Valve_105", "Valve_x.Valve_106", "Valve_x.Valve_107", "Valve_x.Valve_108", "Valve_x.Valve_109", "Valve_x.Valve_110", "Valve_x.Valve_111", "Valve_x.Valve_112", "Valve_x.Valve_113", "Valve_x.Valve_114", "Valve_x.Valve_115", "Valve_x.Valve_116", "Valve_x.Valve_117", "Valve_x.Valve_118", "Valve_x.Valve_119", "Valve_x.Valve_120", "Valve_x.Valve_121", "Valve_x.Valve_122", "Valve_x.Valve_123", "Valve_x.Valve_124", "Valve_x.Valve_125", "Valve_x.Valve_126", "Valve_x.Valve_127"]
  in  "Valve":bool[](array[boolean])
  in  "MFC Array":T5[](array[typedef]) {"SetPoint (SCCM)" format="%#.3g"; "Flow (SCCM)" format="%#.4g"}
  in  "PC Array":T6[](array[typedef])
  in  "RTPC Array":T7[](array[typedef])
  out "GP275 Array":T8[](array[typedef])
  in  "GP354":T9
  in  "BAR Array":T10[](array[typedef])
  in  "EZ-ZONE Output Cluster":T11={"Loop Control Mode"=10, "Closed Loop Set Point"=75.0, "Open Loop Set Point"=0.0, "Alarm 1 - High Set Point"=150.0, "Alarm 1 - Low Set Point"=0.0, "Alarm 2 - High Set Point"=150.0, "Alarm 2 - Low Set Point"=0.0, "Alarm 3 - High Set Point"=150.0, "Alarm 3 - Low Set Point"=0.0, "Alarm 4 - High Set Point"=150.0, "Alarm 4 - Low Set Point"=0.0, "Profile Action Request"=61, "Profile Start"=0, "Heat Proportional Band"=14.0, "Cool Proportional Band"=14.0, "Time Integral"=180.0, "Time Derivative"=0.0, "Heat Hysteresis"=2.0, "Cool Hysteresis"=2.0, "Dead Band"=0.0} {"Profile Action Request" items=["None"=61, "Start a Profile"=196, "Start a Step"=89, "Pause"=146, "Resume"=147, "End"=148]; "Loop Control Mode" items=["Off"=62, "Auto (closed loop)"=10, "Manual (open loop)"=54]}
  in  "EZ-ZONE Input Cluster":T12={"Device Status"=0, "Analog Input Value 1"=0.0, "Analog Input Value 2"=0.0, "Heat Power"=0.0, "Cool Power"=0.0, "Profile Start"=0, "Current Profile"=0, "Current Step"=0, "Active Set Point"=0.0, "Step Time Remaining"=0, "Analog Input Error 1"=61, "Analog Input Error 2"=61, "Alarm State 1"=61, "Alarm State 2"=61, "Alarm State 3"=61, "Alarm State 4"=61, "Digital Input Status 5"=41, "Digital Input Status 6"=41, "Control Mode Active"=62, "Limit State"=62, "Profile Action Request"=61} {"Profile Action Request" items=["None"=61, "Start a Profile"=196, "Start a Step"=89, "Pause"=146, "Resume"=147, "End"=148]; "Limit State" items=["Off"=62, "None"=61, "Limit High"=51, "Limit Low"=52, "Error"=28]; "Control Mode Active" items=["Off"=62, "Auto"=10, "Manual"=54]; "Digital Input Status 6" items=["Inactive"=41, "Active"=5]; "Digital Input Status 5" items=["Inactive"=41, "Active"=5]; "Alarm State 4" items=["Startup"=88, "None"=61, "Blocked"=12, "Alarm Low"=8, "Alarm High"=7, "Error"=28]; "Alarm State 3" items=["Startup"=88, "None"=61, "Blocked"=12, "Alarm Low"=8, "Alarm High"=7, "Error"=28]; "Alarm State 2" items=["Startup"=88, "None"=61, "Blocked"=12, "Alarm Low"=8, "Alarm High"=7, "Error"=28]; "Alarm State 1" items=["Startup"=88, "None"=61, "Blocked"=12, "Alarm Low"=8, "Alarm High"=7, "Error"=28]; "Analog Input Error 2" items=["None"=61, "Open"=65, "Shorted"=127, "Measurement Error"=140, "Bad Calibration Data"=139, "Ambient Error"=9, "RTD Lead Resistance Error"=141]; "Analog Input Error 1" items=["None"=61, "Open"=65, "Shorted"=127, "Measurement Error"=140, "Bad Calibration Data"=139, "Ambient Error"=9, "RTD Lead Resistance Error"=141]}
  in  "Data":u8[](array[numeric])=[0, 0, 0, 0, 0, 0] format="%x"
  in  "TurboMotor Command Cluster":T13={"Enable"=FALSE, "Hard Stop"=FALSE, "Smooth Stop"=FALSE, "Direction"=FALSE, "Incremental"=FALSE, "Load Data/Start Profile"=FALSE, "Axis Number"=0, "Message Type"=0, "Data"=[0, 0, 0, 0, 0, 0]} {"Data" format="%x"}
  out "TurboMotor Response Cluster":T14 {"Data" format="%x"}
  in  "Devices":T15[](array[typedef])=[{"Dnet"="A", "Node"=1, "Type"="MFC", "ID Number"=1, "SCCM"=200.0, "FullScale"=24576.0, "Input Bytes"=8, "Output Bytes"=2, "Input Start Location"=0, "Output Start Location"=0, "Enabled"=TRUE, "Bytes"=[0, 0]}, {"Dnet"="A", "Node"=2, "Type"="MFC", "ID Number"=44, "SCCM"=2000.0, "FullScale"=24576.0, "Input Bytes"=8, "Output Bytes"=2, "Input Start Location"=8, "Output Start Location"=2, "Enabled"=TRUE, "Bytes"=[0, 0]}, {"Dnet"="A", "Node"=3, "Type"="MFC", "ID Number"=45, "SCCM"=200.0, "FullScale"=24576.0, "Input Bytes"=8, "Output Bytes"=2, "Input Start Location"=16, "Output Start Location"=4, "Enabled"=TRUE, "Bytes"=[0, 0]}, {"Dnet"="A", "Node"=4, "Type"="PC", "ID Number"=10, "SCCM"=2000.0, "FullScale"=0.0, "Input Bytes"=8, "Output Bytes"=2, "Input Start Location"=24, "Output Start Location"=6, "Enabled"=TRUE, "Bytes"=[0, 0]}, {"Dnet"="A", "Node"=5, "Type"="MFC", "ID Number"=2, "SCCM"=200.0, "FullScale"=24576.0, "Input Bytes"=8, "Output Bytes"=2, "Input Start Location"=32, "Output Start Location"=8, "Enabled"=TRUE, "Bytes"=[0, 0]}, {"Dnet"="A", "Node"=6, "Type"="MFC", "ID Number"=46, "SCCM"=2000.0, "FullScale"=24576.0, "Input Bytes"=8, "Output Bytes"=2, "Input Start Location"=40, "Output Start Location"=10, "Enabled"=TRUE, "Bytes"=[0, 0]}, {"Dnet"="A", "Node"=7, "Type"="MFC", "ID Number"=47, "SCCM"=200.0, "FullScale"=24576.0, "Input Bytes"=8, "Output Bytes"=2, "Input Start Location"=48, "Output Start Location"=12, "Enabled"=TRUE, "Bytes"=[0, 0]}, {"Dnet"="A", "Node"=8, "Type"="PC", "ID Number"=11, "SCCM"=2000.0, "FullScale"=0.0, "Input Bytes"=8, "Output Bytes"=2, "Input Start Location"=56, "Output Start Location"=14, "Enabled"=TRUE, "Bytes"=[0, 0]}, {"Dnet"="A", "Node"=9, "Type"="MFC", "ID Number"=3, "SCCM"=1000.0, "FullScale"=24576.0, "Input Bytes"=8, "Output Bytes"=2, "Input Start Location"=64, "Output Start Location"=16, "Enabled"=TRUE, "Bytes"=[0, 0]}, {"Dnet"="A", "Node"=10, "Type"="PC", "ID Number"=12, "SCCM"=1000.0, "FullScale"=0.0, "Input Bytes"=8, "Output Bytes"=2, "Input Start Location"=72, "Output Start Location"=18, "Enabled"=TRUE, "Bytes"=[0, 0]}, {"Dnet"="A", "Node"=11, "Type"="UNITMFC", "ID Number"=4, "SCCM"=500.0, "FullScale"=0.0, "Input Bytes"=8, "Output Bytes"=2, "Input Start Location"=80, "Output Start Location"=20, "Enabled"=TRUE, "Bytes"=[0, 0]}, {"Dnet"="A", "Node"=12, "Type"="PC", "ID Number"=13, "SCCM"=500.0, "FullScale"=0.0, "Input Bytes"=8, "Output Bytes"=2, "Input Start Location"=88, "Output Start Location"=22, "Enabled"=TRUE, "Bytes"=[0, 0]}, {"Dnet"="A", "Node"=13, "Type"="MFC", "ID Number"=5, "SCCM"=100.0, "FullScale"=24576.0, "Input Bytes"=8, "Output Bytes"=2, "Input Start Location"=96, "Output Start Location"=24, "Enabled"=TRUE, "Bytes"=[0, 0]}, {"Dnet"="A", "Node"=14, "Type"="MFC", "ID Number"=48, "SCCM"=1000.0, "FullScale"=24576.0, "Input Bytes"=8, "Output Bytes"=2, "Input Start Location"=104, "Output Start Location"=26, "Enabled"=TRUE, "Bytes"=[0, 0]}, {"Dnet"="A", "Node"=15, "Type"="MFC", "ID Number"=49, "SCCM"=100.0, "FullScale"=24576.0, "Input Bytes"=8, "Output Bytes"=2, "Input Start Location"=112, "Output Start Location"=28, "Enabled"=TRUE, "Bytes"=[0, 0]}, {"Dnet"="A", "Node"=16, "Type"="PC", "ID Number"=14, "SCCM"=1000.0, "FullScale"=0.0, "Input Bytes"=8, "Output Bytes"=2, "Input Start Location"=120, "Output Start Location"=30, "Enabled"=TRUE, "Bytes"=[0, 0]}, {"Dnet"="A", "Node"=17, "Type"="MFC", "ID Number"=6, "SCCM"=100.0, "FullScale"=24576.0, "Input Bytes"=8, "Output Bytes"=2, "Input Start Location"=128, "Output Start Location"=32, "Enabled"=TRUE, "Bytes"=[0, 0]}, {"Dnet"="A", "Node"=19, "Type"="MFC", "ID Number"=51, "SCCM"=100.0, "FullScale"=24576.0, "Input Bytes"=8, "Output Bytes"=2, "Input Start Location"=136, "Output Start Location"=34, "Enabled"=TRUE, "Bytes"=[0, 0]}, {"Dnet"="A", "Node"=20, "Type"="PC", "ID Number"=15, "SCCM"=1000.0, "FullScale"=0.0, "Input Bytes"=8, "Output Bytes"=2, "Input Start Location"=144, "Output Start Location"=36, "Enabled"=TRUE, "Bytes"=[0, 0]}, {"Dnet"="A", "Node"=21, "Type"="MFC", "ID Number"=7, "SCCM"=100.0, "FullScale"=24576.0, "Input Bytes"=8, "Output Bytes"=2, "Input Start Location"=152, "Output Start Location"=38, "Enabled"=TRUE, "Bytes"=[0, 0]}, {"Dnet"="A", "Node"=23, "Type"="MFC", "ID Number"=53, "SCCM"=100.0, "FullScale"=24576.0, "Input Bytes"=8, "Output Bytes"=2, "Input Start Location"=160, "Output Start Location"=40, "Enabled"=TRUE, "Bytes"=[0, 0]}, {"Dnet"="A", "Node"=24, "Type"="PC", "ID Number"=16, "SCCM"=1000.0, "FullScale"=0.0, "Input Bytes"=8, "Output Bytes"=2, "Input Start Location"=168, "Output Start Location"=42, "Enabled"=TRUE, "Bytes"=[0, 0]}, {"Dnet"="A", "Node"=25, "Type"="MFC", "ID Number"=8, "SCCM"=200.0, "FullScale"=24576.0, "Input Bytes"=8, "Output Bytes"=2, "Input Start Location"=176, "Output Start Location"=44, "Enabled"=TRUE, "Bytes"=[0, 0]}, {"Dnet"="A", "Node"=27, "Type"="MFC", "ID Number"=55, "SCCM"=200.0, "FullScale"=24576.0, "Input Bytes"=8, "Output Bytes"=2, "Input Start Location"=184, "Output Start Location"=46, "Enabled"=TRUE, "Bytes"=[0, 0]}, {"Dnet"="A", "Node"=28, "Type"="PC", "ID Number"=17, "SCCM"=1000.0, "FullScale"=0.0, "Input Bytes"=8, "Output Bytes"=2, "Input Start Location"=192, "Output Start Location"=48, "Enabled"=TRUE, "Bytes"=[0, 0]}, {"Dnet"="A", "Node"=31, "Type"="MFC", "ID Number"=37, "SCCM"=100.0, "FullScale"=24576.0, "Input Bytes"=8, "Output Bytes"=2, "Input Start Location"=200, "Output Start Location"=50, "Enabled"=TRUE, "Bytes"=[0, 0]}, {"Dnet"="A", "Node"=32, "Type"="MFC", "ID Number"=56, "SCCM"=500.0, "FullScale"=24576.0, "Input Bytes"=8, "Output Bytes"=2, "Input Start Location"=208, "Output Start Location"=52, "Enabled"=TRUE, "Bytes"=[0, 0]}, {"Dnet"="A", "Node"=37, "Type"="MFC", "ID Number"=52, "SCCM"=1000.0, "FullScale"=24576.0, "Input Bytes"=8, "Output Bytes"=2, "Input Start Location"=216, "Output Start Location"=54, "Enabled"=TRUE, "Bytes"=[0, 0]}, {"Dnet"="A", "Node"=42, "Type"="MFC", "ID Number"=42, "SCCM"=500.0, "FullScale"=24576.0, "Input Bytes"=8, "Output Bytes"=2, "Input Start Location"=224, "Output Start Location"=56, "Enabled"=TRUE, "Bytes"=[0, 0]}, {"Dnet"="A", "Node"=48, "Type"="BAR", "ID Number"=90, "SCCM"=0.0, "FullScale"=0.0, "Input Bytes"=3, "Output Bytes"=0, "Input Start Location"=232, "Output Start Location"=58, "Enabled"=TRUE, "Bytes"=[]}, {"Dnet"="A", "Node"=49, "Type"="RTPC", "ID Number"=29, "SCCM"=5000.0, "FullScale"=24576.0, "Input Bytes"=8, "Output Bytes"=3, "Input Start Location"=235, "Output Start Location"=58, "Enabled"=TRUE, "Bytes"=[0, 0, 0]}, {"Dnet"="A", "Node"=50, "Type"="UNITMFC", "ID Number"=50, "SCCM"=1000.0, "FullScale"=24576.0, "Input Bytes"=8, "Output Bytes"=2, "Input Start Location"=243, "Output Start Location"=61, "Enabled"=TRUE, "Bytes"=[0, 0]}, {"Dnet"="A", "Node"=51, "Type"="UNITMFC", "ID Number"=54, "SCCM"=2000.0, "FullScale"=24576.0, "Input Bytes"=8, "Output Bytes"=2, "Input Start Location"=251, "Output Start Location"=63, "Enabled"=TRUE, "Bytes"=[0, 0]}, {"Dnet"="A", "Node"=53, "Type"="RTPC", "ID Number"=27, "SCCM"=5000.0, "FullScale"=24576.0, "Input Bytes"=8, "Output Bytes"=3, "Input Start Location"=259, "Output Start Location"=65, "Enabled"=TRUE, "Bytes"=[0, 0, 0]}, {"Dnet"="A", "Node"=54, "Type"="RTPC", "ID Number"=28, "SCCM"=5000.0, "FullScale"=24576.0, "Input Bytes"=8, "Output Bytes"=3, "Input Start Location"=267, "Output Start Location"=68, "Enabled"=TRUE, "Bytes"=[0, 0, 0]}, {"Dnet"="A", "Node"=55, "Type"="MFC", "ID Number"=57, "SCCM"=1000.0, "FullScale"=24576.0, "Input Bytes"=8, "Output Bytes"=2, "Input Start Location"=275, "Output Start Location"=71, "Enabled"=TRUE, "Bytes"=[0, 0]}, {"Dnet"="A", "Node"=56, "Type"="MFC", "ID Number"=41, "SCCM"=10.0, "FullScale"=24576.0, "Input Bytes"=8, "Output Bytes"=2, "Input Start Location"=283, "Output Start Location"=73, "Enabled"=TRUE, "Bytes"=[0, 0]}, {"Dnet"="A", "Node"=61, "Type"="BAR", "ID Number"=91, "SCCM"=0.0, "FullScale"=0.0, "Input Bytes"=3, "Output Bytes"=0, "Input Start Location"=291, "Output Start Location"=75, "Enabled"=TRUE, "Bytes"=[]}, {"Dnet"="B", "Node"=1, "Type"="MFC", "ID Number"=78, "SCCM"=2000.0, "FullScale"=24576.0, "Input Bytes"=8, "Output Bytes"=2, "Input Start Location"=294, "Output Start Location"=75, "Enabled"=TRUE, "Bytes"=[0, 0]}, {"Dnet"="B", "Node"=2, "Type"="MFC", "ID Number"=79, "SCCM"=2000.0, "FullScale"=24576.0, "Input Bytes"=8, "Output Bytes"=2, "Input Start Location"=302, "Output Start Location"=77, "Enabled"=TRUE, "Bytes"=[0, 0]}, {"Dnet"="B", "Node"=3, "Type"="MFC", "ID Number"=80, "SCCM"=2000.0, "FullScale"=24576.0, "Input Bytes"=8, "Output Bytes"=2, "Input Start Location"=310, "Output Start Location"=79, "Enabled"=TRUE, "Bytes"=[0, 0]}, {"Dnet"="B", "Node"=4, "Type"="MFC", "ID Number"=83, "SCCM"=20000.0, "FullScale"=24576.0, "Input Bytes"=8, "Output Bytes"=2, "Input Start Location"=318, "Output Start Location"=81, "Enabled"=TRUE, "Bytes"=[0, 0]}, {"Dnet"="B", "Node"=5, "Type"="MFC", "ID Number"=81, "SCCM"=20000.0, "FullScale"=24576.0, "Input Bytes"=8, "Output Bytes"=2, "Input Start Location"=326, "Output Start Location"=83, "Enabled"=TRUE, "Bytes"=[0, 0]}, {"Dnet"="B", "Node"=6, "Type"="MFC", "ID Number"=82, "SCCM"=20000.0, "FullScale"=24576.0, "Input Bytes"=8, "Output Bytes"=2, "Input Start Location"=334, "Output Start Location"=85, "Enabled"=TRUE, "Bytes"=[0, 0]}, {"Dnet"="B", "Node"=8, "Type"="MFC", "ID Number"=68, "SCCM"=2000.0, "FullScale"=24576.0, "Input Bytes"=8, "Output Bytes"=2, "Input Start Location"=342, "Output Start Location"=87, "Enabled"=TRUE, "Bytes"=[0, 0]}, {"Dnet"="B", "Node"=9, "Type"="MFC", "ID Number"=85, "SCCM"=1000.0, "FullScale"=24576.0, "Input Bytes"=8, "Output Bytes"=2, "Input Start Location"=350, "Output Start Location"=89, "Enabled"=TRUE, "Bytes"=[0, 0]}, {"Dnet"="B", "Node"=10, "Type"="MFC", "ID Number"=69, "SCCM"=2000.0, "FullScale"=24576.0, "Input Bytes"=8, "Output Bytes"=2, "Input Start Location"=358, "Output Start Location"=91, "Enabled"=TRUE, "Bytes"=[0, 0]}, {"Dnet"="B", "Node"=11, "Type"="MFC", "ID Number"=86, "SCCM"=2000.0, "FullScale"=24576.0, "Input Bytes"=8, "Output Bytes"=2, "Input Start Location"=366, "Output Start Location"=93, "Enabled"=TRUE, "Bytes"=[0, 0]}, {"Dnet"="B", "Node"=12, "Type"="MFC", "ID Number"=70, "SCCM"=500.0, "FullScale"=24576.0, "Input Bytes"=8, "Output Bytes"=2, "Input Start Location"=374, "Output Start Location"=95, "Enabled"=TRUE, "Bytes"=[0, 0]}, {"Dnet"="B", "Node"=13, "Type"="MFC", "ID Number"=73, "SCCM"=1000.0, "FullScale"=24576.0, "Input Bytes"=8, "Output Bytes"=2, "Input Start Location"=382, "Output Start Location"=97, "Enabled"=TRUE, "Bytes"=[0, 0]}, {"Dnet"="B", "Node"=14, "Type"="MFC", "ID Number"=74, "SCCM"=1000.0, "FullScale"=24576.0, "Input Bytes"=8, "Output Bytes"=2, "Input Start Location"=390, "Output Start Location"=99, "Enabled"=TRUE, "Bytes"=[0, 0]}, {"Dnet"="B", "Node"=15, "Type"="MFC", "ID Number"=75, "SCCM"=5000.0, "FullScale"=24576.0, "Input Bytes"=8, "Output Bytes"=2, "Input Start Location"=398, "Output Start Location"=101, "Enabled"=TRUE, "Bytes"=[0, 0]}, {"Dnet"="B", "Node"=16, "Type"="BAR", "ID Number"=92, "SCCM"=0.0, "FullScale"=0.0, "Input Bytes"=3, "Output Bytes"=0, "Input Start Location"=406, "Output Start Location"=103, "Enabled"=TRUE, "Bytes"=[]}, {"Dnet"="B", "Node"=21, "Type"="GP354", "ID Number"=0, "SCCM"=0.0, "FullScale"=0.0, "Input Bytes"=3, "Output Bytes"=1, "Input Start Location"=409, "Output Start Location"=103, "Enabled"=TRUE, "Bytes"=[0]}, {"Dnet"="B", "Node"=22, "Type"="GP275", "ID Number"=0, "SCCM"=0.0, "FullScale"=0.0, "Input Bytes"=5, "Output Bytes"=0, "Input Start Location"=412, "Output Start Location"=104, "Enabled"=TRUE, "Bytes"=[]}, {"Dnet"="C", "Node"=1, "Type"="FESTO", "ID Number"=1, "SCCM"=0.0, "FullScale"=0.0, "Input Bytes"=2, "Output Bytes"=2, "Input Start Location"=417, "Output Start Location"=104, "Enabled"=TRUE, "Bytes"=[0, 0]}, {"Dnet"="C", "Node"=2, "Type"="FESTO", "ID Number"=2, "SCCM"=0.0, "FullScale"=0.0, "Input Bytes"=2, "Output Bytes"=2, "Input Start Location"=419, "Output Start Location"=106, "Enabled"=TRUE, "Bytes"=[0, 0]}, {"Dnet"="C", "Node"=3, "Type"="FESTO", "ID Number"=3, "SCCM"=0.0, "FullScale"=0.0, "Input Bytes"=2, "Output Bytes"=2, "Input Start Location"=421, "Output Start Location"=108, "Enabled"=TRUE, "Bytes"=[0, 0]}, {"Dnet"="C", "Node"=4, "Type"="FESTO", "ID Number"=4, "SCCM"=0.0, "FullScale"=0.0, "Input Bytes"=2, "Output Bytes"=2, "Input Start Location"=423, "Output Start Location"=110, "Enabled"=TRUE, "Bytes"=[0, 0]}, {"Dnet"="C", "Node"=5, "Type"="FESTO", "ID Number"=5, "SCCM"=0.0, "FullScale"=0.0, "Input Bytes"=2, "Output Bytes"=2, "Input Start Location"=425, "Output Start Location"=112, "Enabled"=TRUE, "Bytes"=[0, 0]}, {"Dnet"="C", "Node"=6, "Type"="FESTO", "ID Number"=6, "SCCM"=0.0, "FullScale"=0.0, "Input Bytes"=2, "Output Bytes"=2, "Input Start Location"=427, "Output Start Location"=114, "Enabled"=TRUE, "Bytes"=[0, 0]}, {"Dnet"="C", "Node"=7, "Type"="FESTO", "ID Number"=7, "SCCM"=0.0, "FullScale"=0.0, "Input Bytes"=2, "Output Bytes"=2, "Input Start Location"=429, "Output Start Location"=116, "Enabled"=TRUE, "Bytes"=[0, 0]}, {"Dnet"="C", "Node"=8, "Type"="FESTO", "ID Number"=8, "SCCM"=0.0, "FullScale"=0.0, "Input Bytes"=2, "Output Bytes"=2, "Input Start Location"=431, "Output Start Location"=118, "Enabled"=TRUE, "Bytes"=[0, 0]}]
  in  "Stop":bool
  # "GET attribute"
  # "SET attribute"
  # "Data Low Byte"
  # "Middle Low Byte"
  # "Middle High Byte"
  # "Data High Byte"
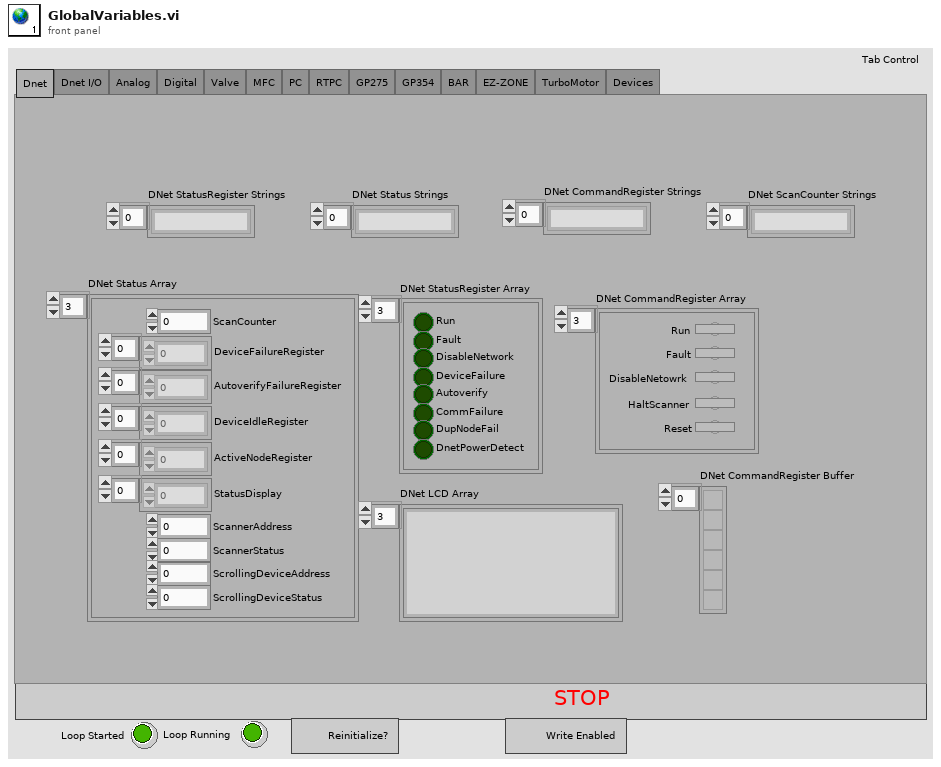
[diagram p1: front panel]
types:
  T1 = enum32{"Dnet", "Dnet I/O", "Analog", "Digital", "Valve", "MFC", "PC", "RTPC", "GP275", "GP354", "BAR", "EZ-ZONE", "TurboMotor", "Devices"}
  T2 = typedef "DNet CommandRegister Cluster.ctl" = cluster{"Run":bool, "Fault":bool, "DisableNetowrk":bool, "HaltScanner":bool, "Reset":bool}
  T3 = typedef "DNet Status Cluster.ctl" = cluster{"ScanCounter":u32, "DeviceFailureRegister":u8[], "AutoverifyFailureRegister":u8[], "DeviceIdleRegister":u8[], "ActiveNodeRegister":u8[], "StatusDisplay":u8[], "ScannerAddress":u8, "ScannerStatus":u8, "ScrollingDeviceAddress":u8, "ScrollingDeviceStatus":u8}
  T4 = typedef "DNet StatusRegister Cluster.ctl" = cluster{"Run":bool, "Fault":bool, "DisableNetwork":bool, "DeviceFailure":bool, "Autoverify":bool, "CommFailure":bool, "DupNodeFail":bool, "DnetPowerDetect":bool}
  T5 = typedef "MFC Cluster.ctl" = cluster{"ID Number":u8, "Status":bool[], "Flow (SCCM)":dbl, "SetPoint (SCCM)":dbl, "Actuator Override":i8, "Actuator Drive Valve":i16, "Setpoint Output":dbl}
  T6 = typedef "PC Cluster.ctl" = cluster{"ID Number":u8, "Status":bool[], "Flow (SCCM)":dbl, "SetPoint (SCCM)":dbl, "Actuator Override":i8, "Actuator Drive Valve":i16, "Setpoint Output":dbl}
  T7 = typedef "RTPC Cluster.ctl" = cluster{"ID Number":u8, "Status":bool[], "Flow (SCCM)":dbl, "Pressure (SCCM)":dbl, "Valve":i16, "Active Instance":i8, "Output":dbl}
  T8 = typedef "GP275 Cluster.ctl" = cluster{"Pressure (Torr)":sgl}
  T9 = typedef "GP354 Cluster.ctl" = cluster{"Degas":bool, "Enable Filament 1":bool, "Enable Filament 2":bool, "Medium Emission":bool, "Ion Gauge":bool, "High Emission":bool, "Pressure":dbl}
  T10 = typedef "BAR Cluster.ctl" = cluster{"Pressure":dbl}
  T11 = typedef "EZ-ZONE Output Cluster.ctl" = cluster{"Loop Control Mode":u32, "Closed Loop Set Point":sgl, "Open Loop Set Point":sgl, "Alarm 1 - High Set Point":sgl, "Alarm 1 - Low Set Point":sgl, "Alarm 2 - High Set Point":sgl, "Alarm 2 - Low Set Point":sgl, "Alarm 3 - High Set Point":sgl, "Alarm 3 - Low Set Point":sgl, "Alarm 4 - High Set Point":sgl, "Alarm 4 - Low Set Point":sgl, "Profile Action Request":u32, "Profile Start":u32, "Heat Proportional Band":sgl, "Cool Proportional Band":sgl, "Time Integral":sgl, "Time Derivative":sgl, "Heat Hysteresis":sgl, "Cool Hysteresis":sgl, "Dead Band":sgl}
  T12 = typedef "EZ-ZONE Input Cluster.ctl" = cluster{"Device Status":u32, "Analog Input Value 1":sgl, "Analog Input Value 2":sgl, "Heat Power":sgl, "Cool Power":sgl, "Profile Start":u32, "Current Profile":u32, "Current Step":u32, "Active Set Point":sgl, "Step Time Remaining":u32, "Analog Input Error 1":u32, "Analog Input Error 2":u32, "Alarm State 1":u32, "Alarm State 2":u32, "Alarm State 3":u32, "Alarm State 4":u32, "Digital Input Status 5":u32, "Digital Input Status 6":u32, "Control Mode Active":u32, "Limit State":u32, "Profile Action Request":u32}
  T13 = typedef "TurboMotor Command Cluster.ctl" = cluster{"Enable":bool, "Hard Stop":bool, "Smooth Stop":bool, "Direction":bool, "Incremental":bool, "Load Data/Start Profile":bool, "Axis Number":u8, "Message Type":u16, "Data":u8[]}
  T14 = typedef "TurboMotor Response Cluster.ctl" = cluster{"Enable":bool, "Index Level":bool, "Current Direction":bool, "General Fault":bool, "Profile in Progress":bool, "Load Complete":bool, "FE Fault":bool, "Rev Limit":bool, "Fwd Limit":bool, "Axis Number":u8, "Message Type":u16, "Data":u8[]}
  T15 = typedef "Device Cluster.ctl" = cluster{"Dnet":string, "Node":i32, "Type":string, "ID Number":u8, "SCCM":dbl, "FullScale":dbl, "Input Bytes":i32, "Output Bytes":i32, "Input Start Location":i32, "Output Start Location":i32, "Enabled":bool, "Bytes":u8[]}
diagram:
